vi "Test SyncStart 1.vi"() -> ()   [LabVIEW 2017]
uses:
  a7600bc9-169c-437f-81c8-f6caaca9cee6.vi
  fa2ffee0-bbcc-4995-9eb6-2b9b7482cc26.vi
  a5c42a9f-df24-4927-b42d-e4e89422ba5a.vi
  Synchronization/SyncStart/_Obtain SyncStart Queue.vi
panel:
  in  "inited":bool
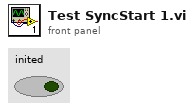
[diagram p1: front panel]
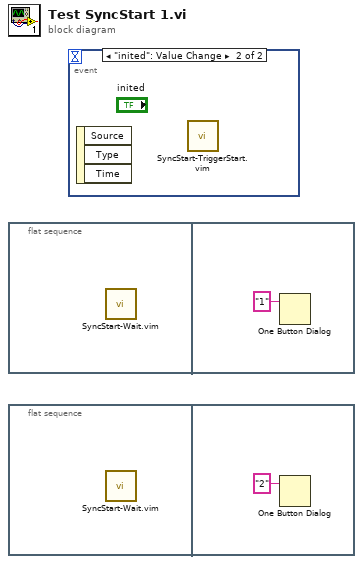
[diagram p0: block diagram]
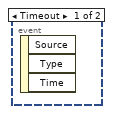
[diagram p2: hidden frame]
diagram:
  n1 = flat-sequence {
    frame #0 {
      n2 = call "SyncStart-Wait.vim"() -> ()  [unwired: 11 in, 1 out]
    }
    frame #1 {
      n3 = One Button Dialog(message="1") -> ()  [unwired: 1 in, 1 out]
    }
  }
  n4 = flat-sequence {
    frame #0 {
      n5 = call "SyncStart-Wait.vim"() -> ()  [unwired: 11 in, 1 out]
    }
    frame #1 {
      n6 = One Button Dialog(message="2") -> ()  [unwired: 1 in, 1 out]
    }
  }
  n7 = event shown="[1] \"inited\": Value Change" {
    selector: _ -> [_ _]
    dyn-events: _ -> [_ _]
    timeout: _ -> [_ _]
    event Timeout {
      n8 = event-data() -> ()  [unwired: 1 in, 3 out]
    }
    event "inited": Value Change {
      n9 = event-data() -> ()  [unwired: 1 in, 3 out]
      n10 = call "SyncStart-TriggerStart.vim"() -> ()  [unwired: 11 in, 1 out]
    }
  }
